vi "Read Manifold Channel Other.vi"(8 "error in":errorcluster, 10 "Manifold Channel Type":T1, 11 "Config Manager in":refnum<class "Config Manager Class.lvclass">) -> (0 "error out":errorcluster, 2 "Channel":i32, 3 "Config Manager out":refnum<class "Config Manager Class.lvclass">)   [LabVIEW 2011, in "Config Manager Class.lvclass"]
uses:
  Config Manager Class.lvclass
  Type Definitions/Manifold Channel Types.ctl
  Config Manager Class.lvclass/Config Manager Class.ctl
  <vilib>/Utility/config.llb/Read Key (I32).vi
  <vilib>/Utility/config.llb/NI_LVConfig.lvlib
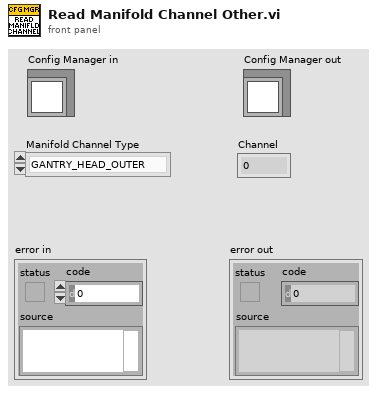
[diagram p1: front panel]
types:
  T1 = typedef "Manifold Channel Types.ctl" = enum16{"GANTRY_HEAD_OUTER", "GANTRY_HEAD_INNER", "GLUE_RESERVOIR_CHUCK", "STAMP_TOOL_CHUCK", "WEIGHT_TOOL_CHUCK"}
  T2 = typedef "NI_LVConfig.lvlib/Config Data RefNum.ctl" = refnum<k1>
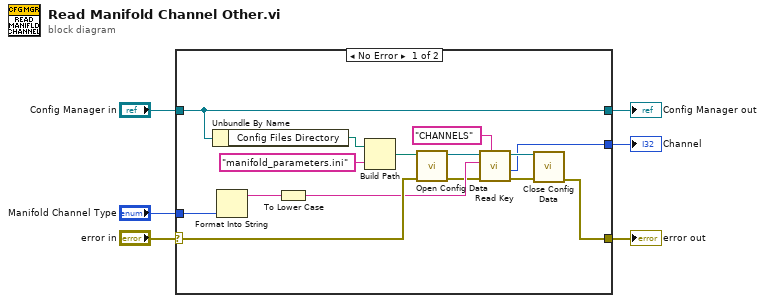
[diagram p0: block diagram]
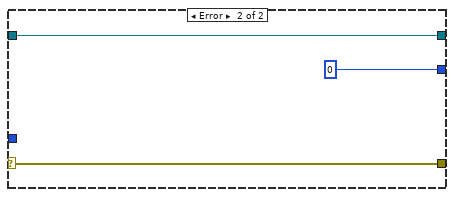
[diagram p2: hidden frame]
diagram:
  n1 = case shown="No Error" "error in" {
    selector: "error in" -> [w16 w24]
    tunnel: [w12 w24] -> w5
    tunnel: [w19 w23] -> w3
    tunnel: "Config Manager in" -> [w19 w23]
    tunnel: [w11 0 ("value")] -> w2
    tunnel: "Manifold Channel Type" -> [w10 _]
    frame No Error {
      n2 = Unbundle By Name(w19) -> ("Config Files Directory"=w18:path)
      n3 = Format Into String(w10) -> (resulting string=w9:string)  [unwired: 3 in, 1 out]
      n4 = To Lower Case(string=w9) -> (all lower case string=w8:string)
      n5 = Build Path(base path=w18, name or relative path="manifold_parameters.ini") -> (appended path=w17:path)
      n6 = call <vilib>:"Open Config Data.vi"("error in (no error)"=w16, "configuration file path"=w17) -> ("error out"=w7:errorcluster, "refnum"=w15:T2)  [unwired: 7 in, 1 out]
      n7 = call-poly <vilib>:"Read Key.vi"("section"="CHANNELS", "error in (no error)"=w7, "key"=w8, "refnum"=w15) -> ("error out"=w13:errorcluster, "value"=w11:i32, "refnum out"=w14:T2)  [unwired: 4 in, 1 out]
      n8 = call <vilib>:"Close Config Data.vi"("error in (no error)"=w13, "refnum"=w14) -> ("error out"=w12:errorcluster)  [unwired: 8 in, 1 out]
    }
    frame Error {
    }
  }
  "error out" <- w5
  "Config Manager out" <- w3
  "Channel" <- w2
